vi "Remove App.vi"(8 "error in (no error)":errorcluster, 10 "App Path":path, 11 "App in":refnum<class "App.lvclass">) -> (0 "error out":errorcluster, 3 "App out":refnum<class "App.lvclass">)   [LabVIEW 2020, in "PicoG-App.lvlib" / "App.lvclass"]
uses:
  App.lvclass
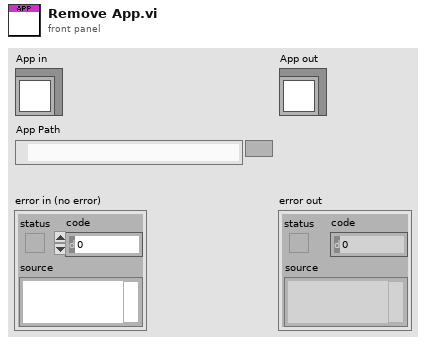
[diagram p1: front panel]
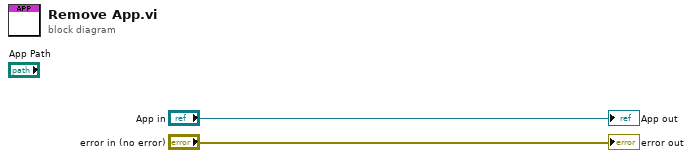
[diagram p0: block diagram]
diagram:
  "error out" <- "error in (no error)"
  "App out" <- "App in"
